vi "read waves - -V1.vi"(11 "file path":path=path "/Users/arkadyshekhter/Library/CloudStorage/Dropbox/shared_AkashAndreas/paper-CeCoIn5-spectroheat/Original RAW data/PLOTME.dat") -> (1 "waves OUT":map{string, dbl[]}(c390))   [LabVIEW 2021]
uses:
  file -- read-write control.ctl
panel:
  out "size(s)":i32
  out "header OUT":string
  out "string array":string[](array[string])
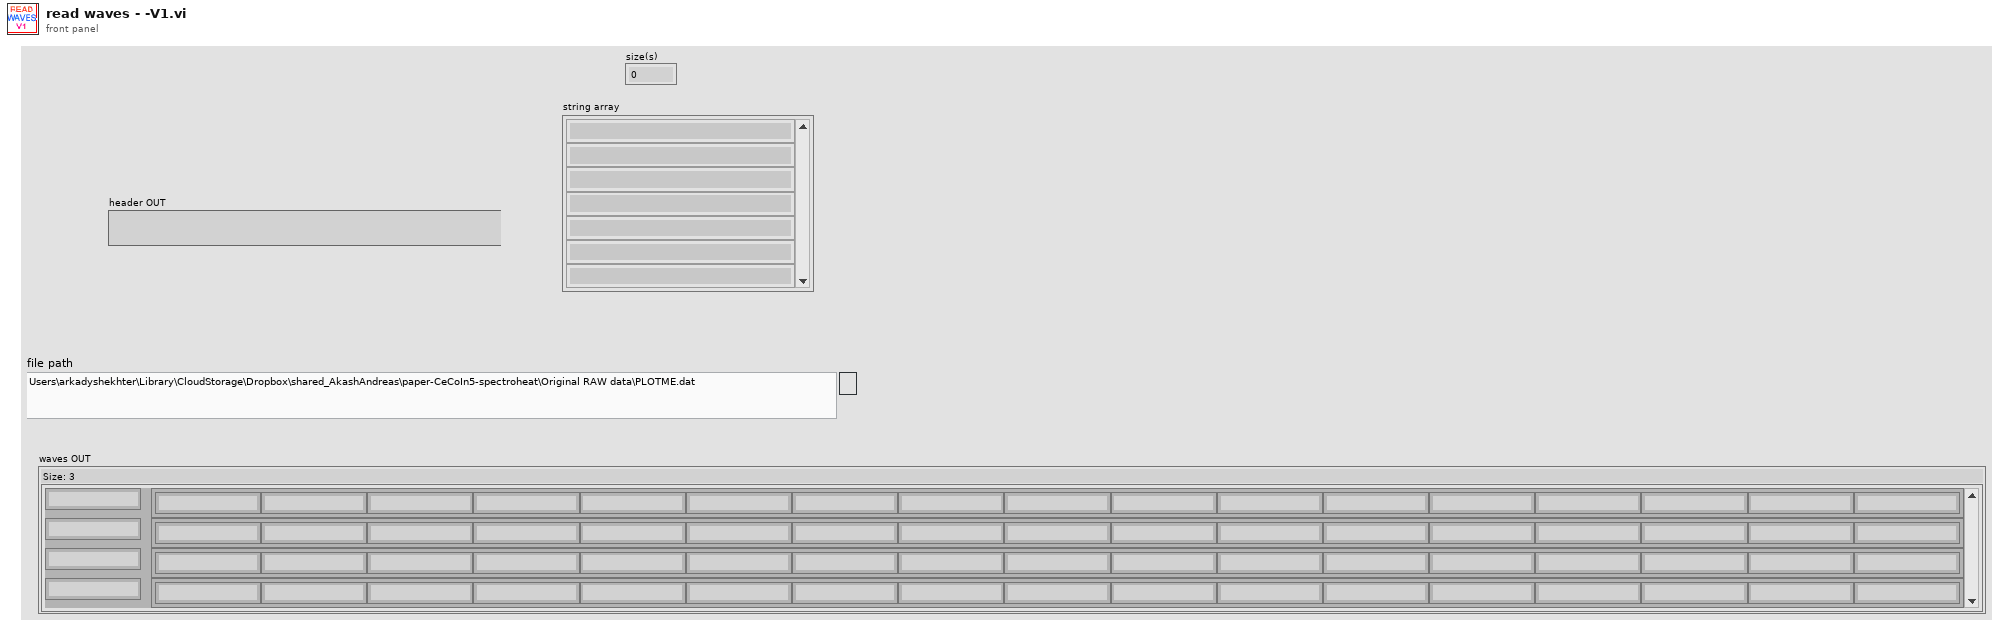
[diagram p1: front panel]
types:
  T1 = typedef "file -- read-write control.ctl" = enum16{"read", "write all", "append one line"}
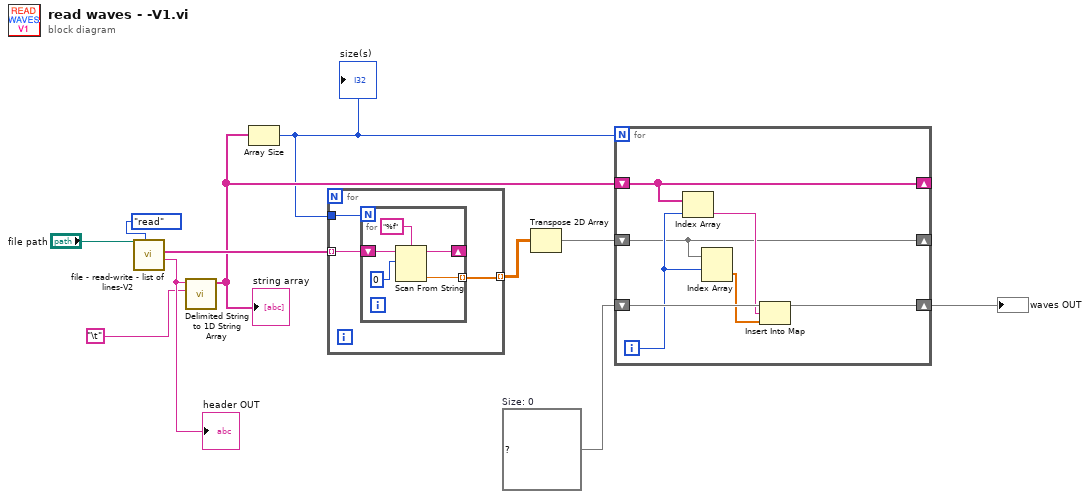
[diagram p0: block diagram]
diagram:
  w7 = map{string, dbl[]} {}  # Size: 0
  n1 = call "file - read-write - list of lines-V2.vi"("read/write control"=file_--_read-write_control."read", "file path"="file path") -> ("header OUT"=w10:string, "list of lines OUT"=w9:string[])  [unwired: 7 in, 1 out]
  "header OUT" <- w10
  n2 = call <vilib>:"Delimited String to 1D String Array.vi"("delimiter"="\t", "delimited string"=w10) -> ("string array"=w3:string[])  [unwired: 9 in]
  "string array" <- w3
  n3 = Array Size(array=w3) -> (size(s)=w2:i32)
  "size(s)" <- w2
  n4 = for {
    tunnel: w9 -> [w14] mode=indexing
    tunnel: [w13] -> w8 mode=indexing
    tunnel: w2 -> [w12]
    n5 = for {
      N: w12 -> [_]
      shift-right: [w16] -> _
      shift-left: w14 -> [w17]
      tunnel: [w15] -> w13 mode=indexing
      n6 = Scan From String(format string="%f", input string=w17, initial scan location=u32 0) -> (remaining string=w16:string, output 1=w15:dbl)  [unwired: 2 in, 2 out]
    }
  }
  n7 = Transpose 2D Array(2D array=w8) -> (transposed array=w4:dbl[][])
  n8 = for {
    N: w2 -> [_]
    shift-right: [w25] -> w5
    shift-left: w7 -> [w26]
    shift-right: [w21] -> _
    shift-left: w4 -> [w21]
    shift-right: [w20] -> _
    shift-left: w3 -> [w20]
    i -> [w24]
    n9 = Index Array(array=w20, index=w24) -> (element=w23:string)
    n10 = Index Array(array=w21, index (row)=w24) -> (element=w22:dbl[])  [unwired: 1 in]
    n11 = Insert Into Map(map in=w26, key=w23, value=w22) -> (map out=w25:map{string, dbl[]})  [unwired: 2 out]
  }
  "waves OUT" <- w5
